vi "Load Player Types.vi"(8 "error in":errorcluster, 11 "Reversi in":refnum<class "Reversi.lvclass">) -> (0 "error out":errorcluster, 3 "Reversi out":refnum<class "Reversi.lvclass">)   [LabVIEW 2020, in "Reversi.lvlib" / "Reversi.lvclass"]
uses:
  Reversi.lvclass
  Player/Player.lvclass
  Human/Human.lvclass
  C:/dev/SoL/summer-of-labview-reversi/Reversi/Player/Player.lvclass
  C:/dev/SoL/summer-of-labview-reversi/Reversi/Human/Human.lvclass
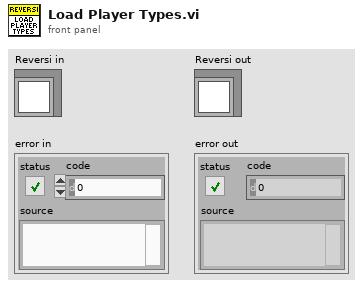
[diagram p1: front panel]
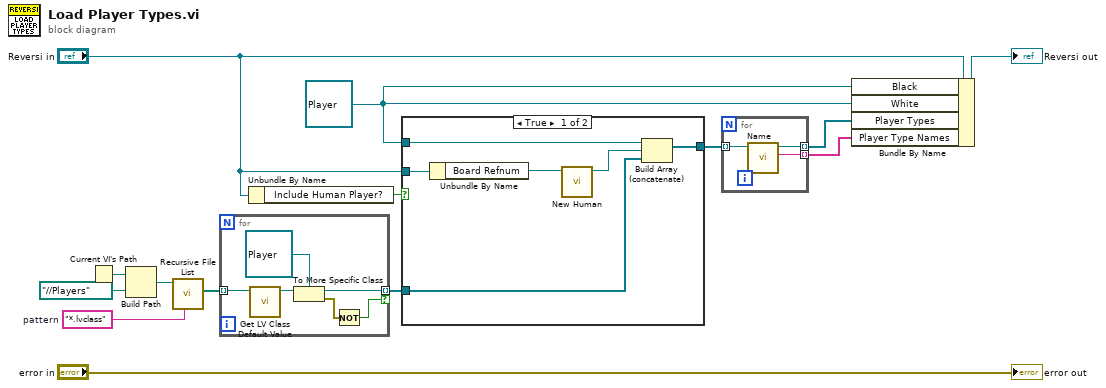
[diagram p0: block diagram]
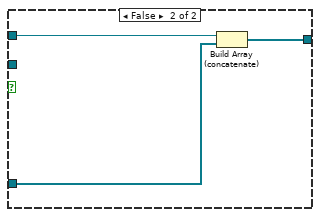
[diagram p2: hidden frame]
diagram:
  w5 = "*.lvclass"  # pattern
  w11 = refnum<class "Player.lvclass"> refnum ("Player")
  n1 = Current VI's Path() -> (path=w7:path)
  n2 = Build Path(base path=w7, name or relative path=path "../../Players" ("Players")) -> (appended path=w6:path)
  n3 = call <vilib>:"Recursive File List.vi"("pattern"=w5, "Folder Path"=w6) -> ("All Files in Dir"=w4:path[])  [unwired: 5 in, 4 out]
  n4 = for {
    tunnel: w4 -> [w19] mode=indexing
    tunnel: [w16] -> w3 mode=indexing if=w15
    n5 = call <vilib>:"Get LV Class Default Value.vi"("class path"=w19) -> ("object"=w18:refnum<class>)  [unwired: 9 in, 1 out]
    n6 = To More Specific Class(target class=refnum<class "Player.lvclass"> refnum ("Player"), reference=w18) -> (specific class reference=w16:refnum<class "Player.lvclass">, error out=w20:errorcluster)  [unwired: 1 in]
    n7 = Not(x=w20) -> (.not. x?=w15:bool)
  }
  n8 = Unbundle By Name("Reversi in") -> ("Include Human Player?"=w2:bool)
  n9 = case shown="True" w2 {
    tunnel: [w26 w29] -> w13
    tunnel: w11 -> [w25 w28]
    tunnel: w3 -> [w24 w27]
    tunnel: "Reversi in" -> [w22 _]
    frame True {
      n10 = Unbundle By Name(w22) -> ("Board Refnum"=w23:refnum<vi>)
      n11 = call "New Human.vi"("Board Refnum"=w23) -> ("Human out"=w21:refnum<class "Human.lvclass">)  [unwired: 9 in, 1 out]
      n12 = Build Array (concatenate)(w25, w21, w24) -> (w26:refnum<class "Player.lvclass">[])
    }
    frame False {
      n13 = Build Array (concatenate)(w28, w27) -> (w29:refnum<class "Player.lvclass">[])
    }
  }
  n14 = for {
    tunnel: w13 -> [w32] mode=indexing
    tunnel: [w31] -> w10 mode=indexing
    tunnel: [w30] -> w9 mode=indexing
    n15 = call-dynamic "Name.vi"("Player in"=w32) -> ("Name"=w30:string, "Player out"=w31:refnum<class "Player.lvclass">)  [unwired: 8 in, 1 out]
  }
  n16 = Bundle By Name(cluster="Reversi in", "Black"=w11, "White"=w11, "Player Types"=w10, "Player Type Names"=w9) -> (→"Reversi out":refnum<class "Reversi.lvclass">)
  "error out" <- "error in"
